vi "Add Hardware.vi"(0 "Microscope in":refnum<class "Microscope.lvclass">, 5 "Device.lvlib:Device.lvclass":refnum<class "Device.lvclass">, 7 "Setting":T1={"Label"="", "DeviceType"="", "DefaultDevice? (F)"=TRUE, "StartAcquiring? (F)"=TRUE}, 11 "error in (no error)":errorcluster) -> (4 "Microscope out":refnum<class "Microscope.lvclass">, 6 "key already included?":bool, 8 "value unchanged?":bool, 15 "error out":errorcluster)   [LabVIEW 2020, in "Microscope.lvlib" / "Microscope.lvclass"]
uses:
  Microscope.lvclass
  Component/Device/Device/Device.lvclass
  Microscope.lvclass/Microscope.ctl
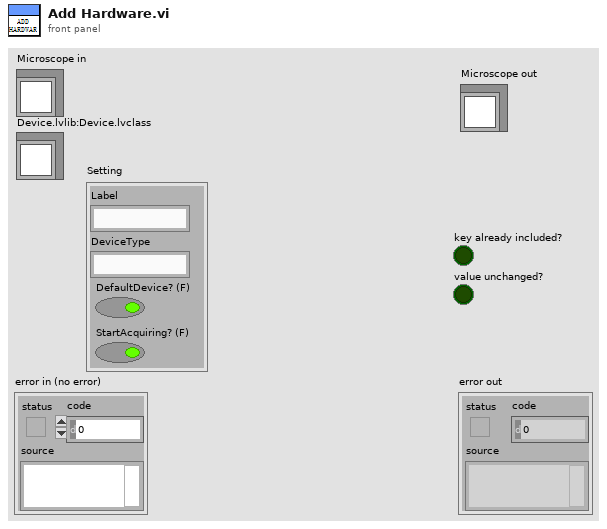
[diagram p1: front panel]
types:
  T1 = cluster{"Label":string, "DeviceType":string, "DefaultDevice? (F)":bool, "StartAcquiring? (F)":bool}
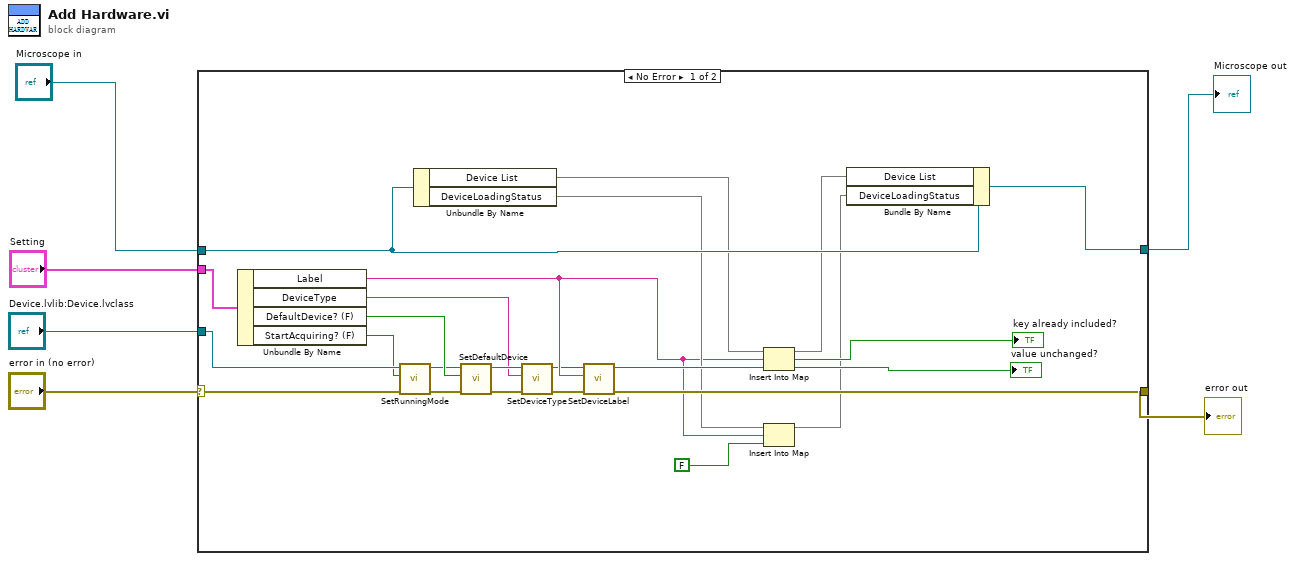
[diagram p0: block diagram]
diagram:
  n1 = case shown="No Error" "error in (no error)" {
    selector: "error in (no error)" -> [w27 w32]
    tunnel: [w26 w32] -> w5
    tunnel: [w23 w31] -> w3
    tunnel: "Microscope in" -> [w30 w31]
    tunnel: "Device.lvlib:Device.lvclass" -> [w17 _]
    tunnel: "Setting" -> [w20 _]
    frame No Error {
      n2 = Unbundle By Name(w20) -> ("Label"=w13:string, "DeviceType"=w7:string, "DefaultDevice? (F)"=w19:bool, "StartAcquiring? (F)"=w15:bool)
      n3 = call-dynamic "SetRunningMode.vi"("error in (no error)"=w27, "RunAfterLoaded?"=w15, "Device in"=w17) -> ("error out"=w18:errorcluster, "Device out"=w16:refnum<class "Device.lvclass">)  [unwired: 7 in]
      n4 = Unbundle By Name(w30) -> ("Device List"=w29:map{string, refnum<class "Device.lvclass">}, "DeviceLoadingStatus"=w14:map{string, bool})
      n5 = call-dynamic "SetDefaultDevice.vi"("error in (no error)"=w18, "DefaultDevice?"=w19, "Device in"=w16) -> ("error out"=w22:errorcluster, "Device out"=w9:refnum<class "Device.lvclass">)  [unwired: 7 in]
      n6 = call-dynamic "SetDeviceType.vi"("error in (no error)"=w22, "Type"=w7, "Device in"=w9) -> ("error out"=w10:errorcluster, "Device out"=w8:refnum<class "Device.lvclass">)  [unwired: 7 in]
      n7 = call-dynamic "SetDeviceLabel.vi"("error in (no error)"=w10, "Label"=w13, "Device in"=w8) -> ("error out"=w26:errorcluster, "Device out"=w21:refnum<class "Device.lvclass">)  [unwired: 7 in]
      n8 = Insert Into Map(map in=w29, key=w13, value=w21) -> (map out=w28:map{string, refnum<class "Device.lvclass">}, key already included?=→"key already included?":bool, value unchanged?=→"value unchanged?":bool)
      n9 = Insert Into Map(map in=w14, key=w13, value=FALSE) -> (map out=w11:map{string, bool})  [unwired: 2 out]
      n10 = Bundle By Name(cluster=w30, "Device List"=w28, "DeviceLoadingStatus"=w11) -> (w23:refnum<class "Microscope.lvclass">)
    }
    frame Error {
    }
  }
  "error out" <- w5
  "Microscope out" <- w3
